vi "niScope Fetch (poly).vi"   [LabVIEW 2011]
doc: "Retrieves data that the digitizer has acquired from a previously initiated acquisition."
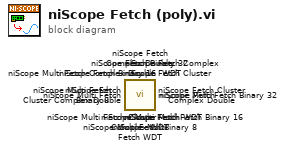
[diagram p0: block diagram]
diagram:
  n1 = call <instrlib>:"niScope Multi Fetch Complex WDT.vi"() -> ()  [unwired: 8 in, 4 out]
  n2 = call <instrlib>:"niScope Fetch Complex WDT.vi"() -> ()  [unwired: 8 in, 4 out]
  n3 = call <instrlib>:"niScope Multi Fetch Cluster Complex Double.vi"() -> ()  [unwired: 8 in, 4 out]
  n4 = call <instrlib>:"niScope Fetch Cluster Complex Double.vi"() -> ()  [unwired: 8 in, 4 out]
  n5 = call <instrlib>:"niScope Multi Fetch Complex Double.vi"() -> ()  [unwired: 8 in, 4 out]
  n6 = call <instrlib>:"niScope Fetch Complex Double.vi"() -> ()  [unwired: 8 in, 4 out]
  n7 = call <instrlib>:"niScope Multi Fetch WDT.vi"() -> ()  [unwired: 8 in, 4 out]
  n8 = call <instrlib>:"niScope Fetch WDT.vi"() -> ()  [unwired: 8 in, 4 out]
  n9 = call <instrlib>:"niScope Multi Fetch.vi"() -> ()  [unwired: 8 in, 4 out]
  n10 = call <instrlib>:"niScope Fetch.vi"() -> ()  [unwired: 8 in, 4 out]
  n11 = call <instrlib>:"niScope Multi Fetch Cluster.vi"() -> ()  [unwired: 8 in, 4 out]
  n12 = call <instrlib>:"niScope Fetch Cluster.vi"() -> ()  [unwired: 8 in, 4 out]
  n13 = call <instrlib>:"niScope Multi Fetch Binary 8.vi"() -> ()  [unwired: 8 in, 4 out]
  n14 = call <instrlib>:"niScope Fetch Binary 32.vi"() -> ()  [unwired: 8 in, 4 out]
  n15 = call <instrlib>:"niScope Multi Fetch Binary 32.vi"() -> ()  [unwired: 8 in, 4 out]
  n16 = call <instrlib>:"niScope Fetch Binary 16.vi"() -> ()  [unwired: 8 in, 4 out]
  n17 = call <instrlib>:"niScope Multi Fetch Binary 16.vi"() -> ()  [unwired: 8 in, 4 out]
  n18 = call <instrlib>:"niScope Fetch Binary 8.vi"() -> ()  [unwired: 8 in, 4 out]
